vi "SMO.ByRefWithEvents.TestLauncher.vi"() -> ()   [LabVIEW 2013, in "SMO.ByRefWithEvents.lvclass"]
doc: "JKI State Machine Objects (SMO) 1.0.0.5\nJKI - JKI\nCopyright (c) 2016, JKI"
uses:
  SMO.ByRefWithEvents.lvclass
  <vilib>/JKI/JKI SMO/SMO/SMO.lvclass
panel:
  in  "Send":bool
  in  "Data":string
  out "error out":errorcluster
  in  "Stop":bool
  # "SMO Test Launcher"
  # "For instructions on how to use the JKI State Machine Objects, examples and video tutorials, visit:\nhttp://jki.net/state-machine-objects/\n\nJKI State Machine Objects™\nhttp://jki.net/state-machine-objects/\nCopyright (C) 2005-2015, JKI <info@jki.net>\nALL RIGHTS RESERVED"
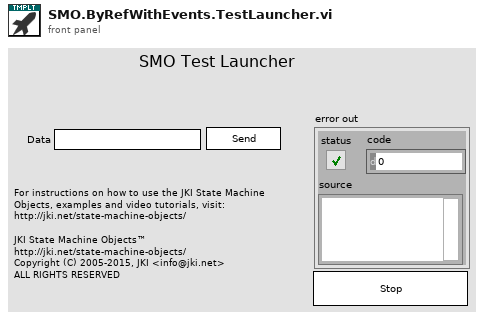
[diagram p1: front panel]
types:
  T1 = cluster{"SMO.Template Public Events":refnum<event-registration>}
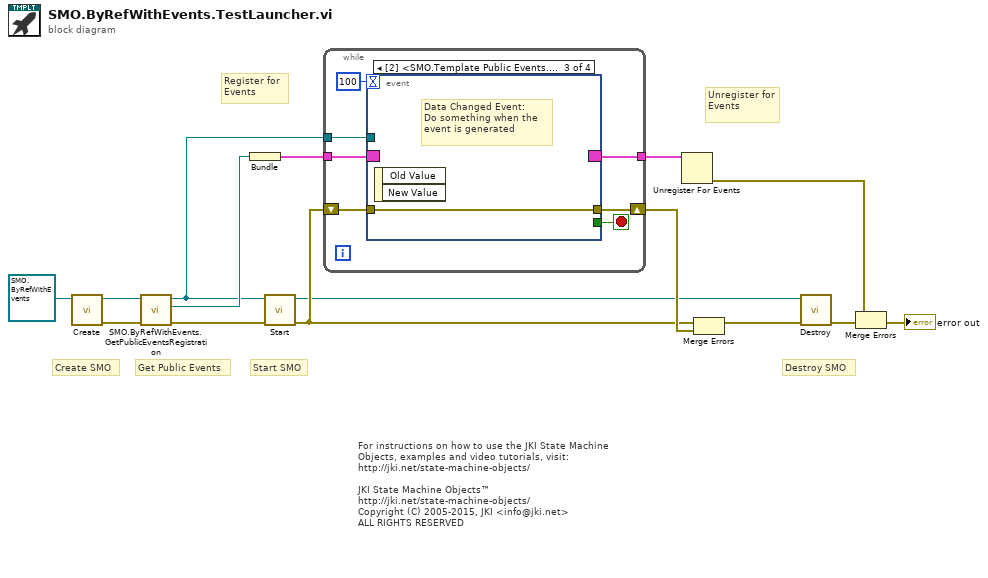
[diagram p0: block diagram]
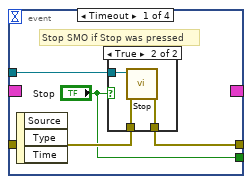
[diagram p2: hidden frame]
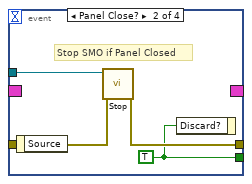
[diagram p4: hidden frame]
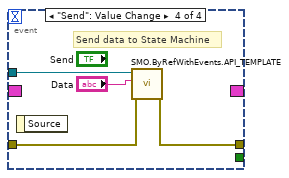
[diagram p5: hidden frame]
diagram:
  # "For instructions on how to use the JKI State Machine Objects, examples and video tutorials, visit:\nhttp://jki.net/state-machine-objects/\n\nJKI State Machine Objects™\nhttp://jki.net/state-machine-objects/\nCopyright (C) 2005-2015, JKI <info@jki.net>\nALL RIGHTS RESERVED"
  # "Get Public Events"
  # "Start SMO"
  # "Destroy SMO"
  # "Create SMO"
  # "Unregister for Events"
  # "Register for Events"
  n1 = call <vilib>:"Create.vi"("SMO"=refnum<class "SMO.ByRefWithEvents.lvclass"> refnum ("SMO.Template.lvclass")) -> ("error out"=w7:errorcluster, "SMO out"=w8:refnum<class "SMO.ByRefWithEvents.lvclass">)  [unwired: 9 in]
  n2 = call "SMO.ByRefWithEvents.GetPublicEventsRegistration.vi"("error in (no error)"=w7, "SMO.ByRefWithEvents"=w8) -> ("error out"=w6:errorcluster, "SMO.Template Public Events"=w5:refnum<event-registration>, "SMO.ByRefWithEvents out"=w2:refnum<class "SMO.ByRefWithEvents.lvclass">)  [unwired: 7 in]
  n3 = Bundle("SMO.Template Public Events"=w5) -> (w14:T1)  [unwired: 1 in]
  n4 = call <vilib>:"Start.vi"("error in (no error)"=w6, "SMO"=w2) -> ("error out"=w4:errorcluster, "SMO out"=w1:refnum<class "SMO.ByRefWithEvents.lvclass">)  [unwired: 8 in]
  n5 = while {
    shift-right: [w21] -> w13
    shift-left: w4 -> [w20]
    tunnel: w14 -> [w19]
    tunnel: [w18] -> w15
    tunnel: w2 -> [w17]
    stop <- w22 stop-if-true
    n6 = event shown="[2] <SMO.Template Public Events.Data Changed>: User Event" {
      selector: w19 -> [_ _ _ _]
      dyn-events: [_ _ _ _] -> w18
      timeout: 100 -> [_ _ _ _]
      tunnel: ["Stop" w31 _ _] -> w22
      tunnel: w17 -> [w26 w34 _ w39]
      tunnel: [w25 w33 w35 w36] -> w21
      tunnel: w20 -> [w24 w32 w35 w37]
      event Timeout {
        # "Stop SMO if Stop was pressed"
        n7 = event-data() -> ()  [unwired: 1 in, 3 out]
        n8 = case shown="True" "Stop" {
          tunnel: w26 -> [_ w30]
          tunnel: [w27 w29] -> w25
          tunnel: w24 -> [w27 w28]
          frame False {
          }
          frame True {
            n9 = call <vilib>:"Stop.vi"("error in (no error)"=w28, "SMO"=w30) -> ("error out"=w29:errorcluster)  [unwired: 8 in, 1 out]
          }
        }
      }
      event Panel Close? {
        w31 = TRUE ("OK")
        # "Stop SMO if Panel Closed"
        n10 = event-data() -> ()  [unwired: 1 in, 1 out]
        n11 = call <vilib>:"Stop.vi"("error in (no error)"=w32, "SMO"=w34) -> ("error out"=w33:errorcluster)  [unwired: 8 in, 1 out]
        n12 = event-data("Discard?"=w31) -> ()  [unwired: 1 in, 1 out]
      }
      event User Event {
        # "Data Changed Event:\nDo something when the\nevent is generated"
        n13 = event-data() -> ()  [unwired: 1 in, 2 out]
      }
      event "Send": Value Change {
        # "Send data to State Machine"
        n14 = event-data() -> ()  [unwired: 1 in, 1 out]
        n15 = call "SMO.ByRefWithEvents.API_TEMPLATE.vi"("error in (no error)"=w37, "myData"="Data", "SMO.ByRefWithEvents"=w39) -> ("error out"=w36:errorcluster)  [unwired: 6 in, 2 out]
      }
    }
  }
  n16 = Unregister For Events(event registration refnum=w15) -> (error out=w12:errorcluster)  [unwired: 1 in]
  n17 = Merge Errors(w4, w13) -> (w3:errorcluster)
  n18 = call <vilib>:"Destroy.vi"("error in (no error)"=w3, "SMO"=w1) -> ("error out"=w10:errorcluster)  [unwired: 9 in]
  n19 = Merge Errors(w12, w10) -> (→"error out":errorcluster)
